vi "Set Panel Initial State.vi"(10 "Title":string, 11 "Main Vi Ref":refnum<vi>) -> (0 "error out":errorcluster)   [LabVIEW 2019, in "Panther Dashboard.lvlib"]
uses:
  Panther Dashboard.lvlib
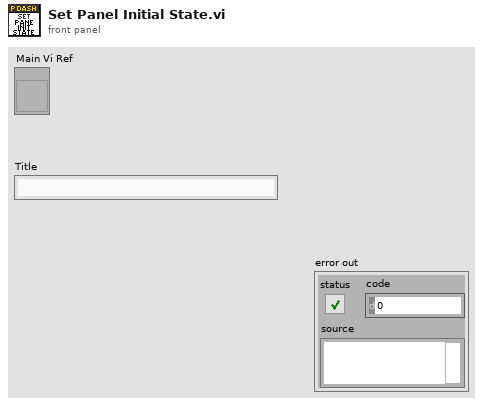
[diagram p1: front panel]
types:
  T1 = enum32{"Invalid", "Standard", "Closed", "Hidden", "Minimized", "Maximized"}
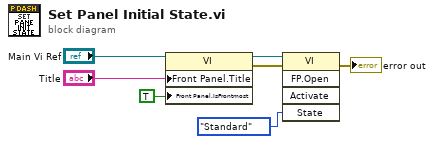
[diagram p0: block diagram]
diagram:
  n1 = property on="Property Node" class="VI"(reference="Main Vi Ref", "Front Panel.Title"="Title", "Front Panel.IsFrontmost"=TRUE ("Front Panel Window:Is Frontmost")) -> (reference out=w2:refnum<vi>, error out=w7:errorcluster)  [unwired: 1 in]
  n2 = invoke on="Invoke Node" class="VI" method="FP.Open"(reference=w2, error in=w7, "State"=T1."Standard") -> (error out=→"error out":errorcluster)  [unwired: 2 in, 4 out]
